vi "Word Clear.vi"(11 "Words_Ref in":refnum<vi>[](array[refnum])) -> (3 "Words_Ref out":refnum<vi>[](array[refnum]))   [LabVIEW 2015]
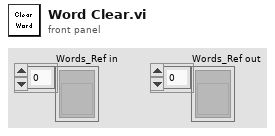
[diagram p1: front panel]
types:
  T1 = enum8{"Enabled", "Disabled", "Disabled and Grayed Out"}
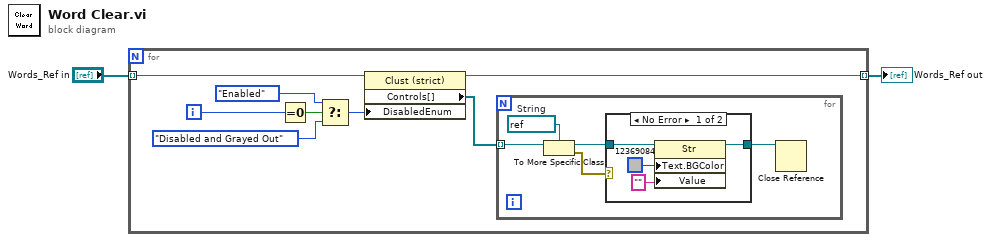
[diagram p0: block diagram]
diagram:
  n1 = for {
    tunnel: "Words_Ref in" -> [w9] mode=indexing
    tunnel: [w3] -> w1 mode=indexing
    i -> [w6]
    n2 = Equal To 0?(x=w6) -> (x = 0?=w7:bool)
    n3 = Select(t=T1."Enabled" ("Disabled"), s=w7, f=T1."Disabled and Grayed Out" ("Disabled")) -> (s? t:f=w8:T1)
    n4 = property class="Clust (strict)"(reference=w9, "DisabledEnum"=w8) -> (reference out=w3:refnum<vi>, "Controls[]"=w10:refnum<vi>[])  [unwired: 1 in, 1 out]
    n5 = for {
      tunnel: w10 -> [w15] mode=indexing
      w13 = refnum<vi> refnum  # String
      n6 = To More Specific Class(target class=w13, reference=w15) -> (specific class reference=w14:refnum<vi>, error out=w12:errorcluster)  [unwired: 1 in]
      n7 = case shown="No Error" w12 {
        tunnel: w14 -> [w19 w20]
        tunnel: [w17 w20] -> w11
        frame No Error {
          n8 = property class="Str"(reference=w19, "Text.BGColor"=u32 12369084, "Value"="") -> (reference out=w17:refnum<vi>)  [unwired: 1 in, 1 out]
        }
        frame Error {
        }
      }
      n9 = Close Reference(reference=w11) -> ()  [unwired: 1 in, 1 out]
    }
  }
  "Words_Ref out" <- w1
